vi "Acquisition_anemometre.vi"() -> (3 "data":u32)   [LabVIEW 2017]
doc: "Ce VI fait l'acquisition de l'anémomètre (entrée compteur)\n\nCopyright | Jixiong Liu & Benoit Mangeard"
uses:
  <vilib>/DAQmx/read.llb/DAQmx Read (Counter U32 1Chan 1Samp).vi
  <vilib>/DAQmx/create/channels.llb/DAQmx Create Channel (CI-Count Edges).vi
  <vilib>/DAQmx/miscellaneous.llb/DAQmx Fill In Error Info.vi
  <resource>/objmgr/daqmx.rc
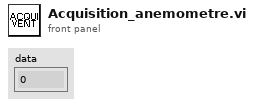
[diagram p1: front panel]
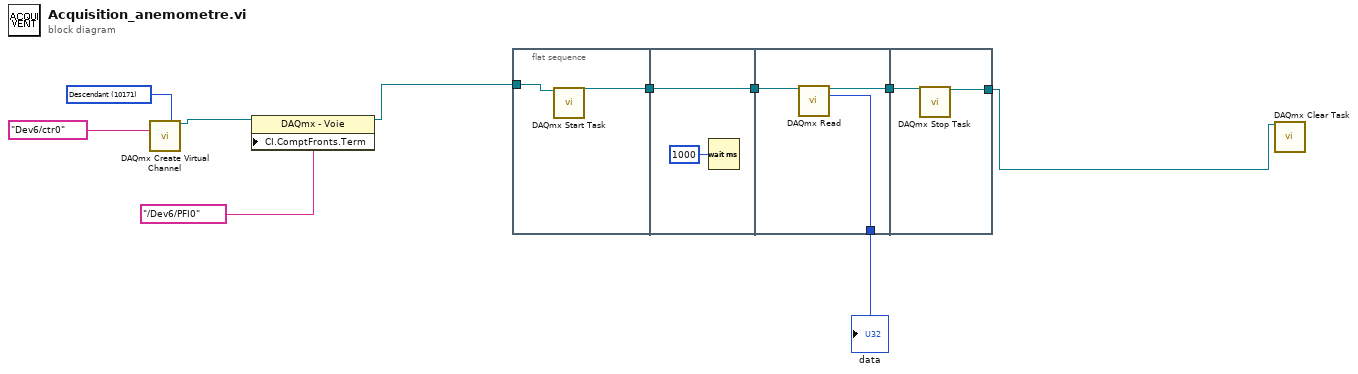
[diagram p0: block diagram]
diagram:
  w1 = 10171 items=["Montant"=10280, "Descendant"=10171] ("edge")
  n1 = call-poly <vilib>:"DAQmx Create Virtual Channel.vi"("edge"=w1, "counter"=tag "Dev6/ctr0") -> ("task out"=w3:refnum<k21>)  [unwired: 12 in, 1 out]
  n2 = property class="DAQmx - Voie"(reference=w3, "CI.ComptFronts.Term"=tag "/Dev6/PFI0") -> (reference out=w6:refnum<k21>)  [unwired: 1 in, 1 out]
  n3 = flat-sequence {
    tunnel: [w12] -> w10
    tunnel: w6 -> [w11]
    tunnel: w10 -> [w13]
    tunnel: [w13] -> w9
    tunnel: [w17] -> w8
    tunnel: [w16] -> w5
    tunnel: w9 -> [w15]
    tunnel: [w19] -> w7
    tunnel: w8 -> [w18]
    frame #0 {
      n4 = call <vilib>:"DAQmx Start Task.vi"("task/channels in"=w11) -> ("task out"=w12:refnum<k21>)  [unwired: 13 in, 1 out]
    }
    frame #1 {
      n5 = Wait (ms)(milliseconds to wait=u32 1000 ("attente (ms)")) -> ()  [unwired: 1 out]
    }
    frame #2 {
      n6 = call-poly <vilib>:"DAQmx Read.vi"("task/channels in"=w15) -> ("task out"=w17:refnum<k21>, "data"=w16:u32)  [unwired: 12 in, 1 out]
    }
    frame #3 {
      n7 = call <vilib>:"DAQmx Stop Task.vi"("task/channels in"=w18) -> ("task out"=w19:refnum<k21>)  [unwired: 13 in, 1 out]
    }
  }
  n8 = call <vilib>:"DAQmx Clear Task.vi"("task in"=w7) -> ()  [unwired: 14 in, 1 out]
  "data" <- w5
